vi "Generate.vi"(8 "error in (no error)":errorcluster, 10 "Coordinates":T1, 11 "Snake in":refnum<class "Snake.lvclass">) -> (0 "error out":errorcluster, 3 "Snake out":refnum<class "Snake.lvclass">)   [LabVIEW 2018, in "Snake.lvclass"]
uses:
  Snake/Snake.lvclass
  Snake/Type Defs/Coordinates.ctl
  Snake/Snake.lvclass/Snake.ctl
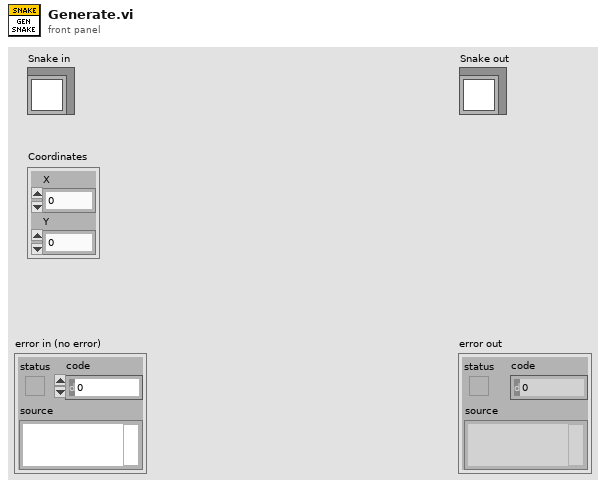
[diagram p1: front panel]
types:
  T1 = typedef "Coordinates.ctl" = cluster{"X":i32, "Y":i32}
  T2 = typedef "Direction.ctl" = enum16{"Up", "Down", "Left", "Right"}
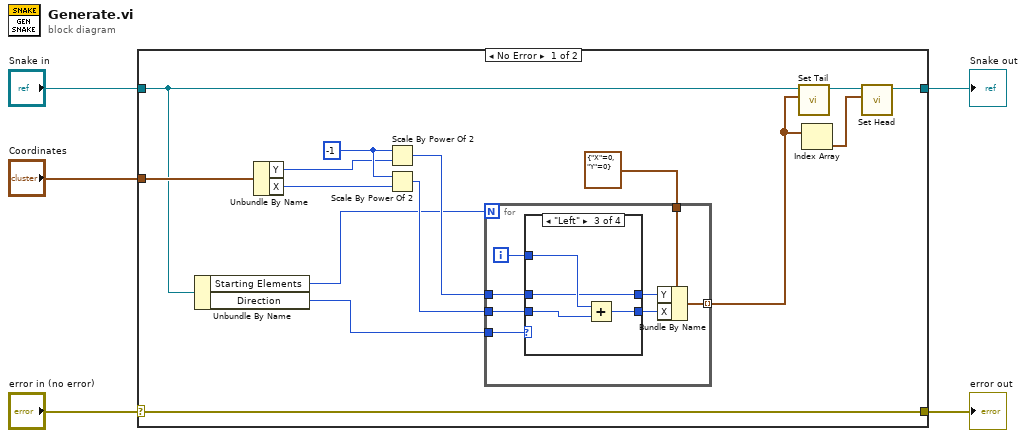
[diagram p0: block diagram]
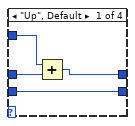
[diagram p2: hidden frame]
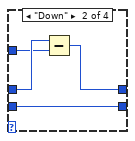
[diagram p3: hidden frame]
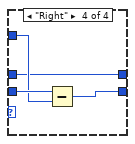
[diagram p4: hidden frame]
diagram:
  n1 = case shown="No Error" "error in (no error)" {
    selector: "error in (no error)" -> [w20 w46]
    tunnel: [w20 w46] -> w4
    tunnel: "Snake in" -> [w6 w45]
    tunnel: [w12 w45] -> w3
    tunnel: "Coordinates" -> [w9 _]
    frame No Error {
      w19 = i16 -1 ("n")
      n2 = Unbundle By Name(w6) -> ("Starting Elements"=w10:i32, "Direction"=w11:T2)
      n3 = Unbundle By Name(w9) -> ("Y"=w7:i32, "X"=w8:i32)
      n4 = Scale By Power Of 2(n=w19, x=w7) -> (x*2^n=w17:i32)
      n5 = Scale By Power Of 2(n=w19, x=w8) -> (x*2^n=w16:i32)
      n6 = for {
        N: w10 -> [_]
        tunnel: T1 {"X"=0, "Y"=0} ("Coordinates") -> [w28]
        tunnel: w17 -> [w25]
        tunnel: w16 -> [w21]
        tunnel: [w27] -> w14 mode=indexing
        tunnel: w11 -> [w26]
        i -> [w24]
        n7 = case shown="\"Left\"" w26 {
          tunnel: w25 -> [w31 w36 w38 w42]
          tunnel: w24 -> [w32 w35 w39 w43]
          tunnel: [w30 w34 w38 w42] -> w23
          tunnel: [w29 w33 w37 w41] -> w22
          tunnel: w21 -> [w29 w33 w40 w44]
          frame "Up", Default {
            n8 = Add(x=w32, y=w31) -> (x+y=w30:i32)
          }
          frame "Down" {
            n9 = Subtract(x=w36, y=w35) -> (x-y=w34:i32)
          }
          frame "Left" {
            n10 = Add(x=w39, y=w40) -> (x+y=w37:i32)
          }
          frame "Right" {
            n11 = Subtract(x=w44, y=w43) -> (x-y=w41:i32)
          }
        }
        n12 = Bundle By Name(cluster=w28, "Y"=w23, "X"=w22) -> (w27:T1)
      }
      n13 = call "Set Tail.vi"("Tail"=w14, "Snake in"=w6) -> ("Snake out"=w15:refnum<class "Snake.lvclass">)  [unwired: 8 in, 1 out]
      n14 = Index Array(array=w14) -> (element=w13:T1)  [unwired: 1 in]
      n15 = call "Set Head.vi"("Coordinates"=w13, "Snake in"=w15) -> ("Snake out"=w12:refnum<class "Snake.lvclass">)  [unwired: 8 in, 1 out]
    }
    frame Error {
    }
  }
  "error out" <- w4
  "Snake out" <- w3
